vi "Data entry form multi-module.vi"(8 "error in (no error)":errorcluster, 9 "Assembly Type":string, 10 "Is Module?":bool, 11 "Database Entry in":refnum<class "Database Entry.lvclass">) -> (0 "error out":errorcluster, 1 "Is Dummy run?":bool, 2 "Aborted":bool, 3 "Database Entry out":refnum<class "Database Entry.lvclass">)   [LabVIEW 2021, in "Database Entry.lvclass"]
uses:
  Database Entry.lvclass
  Database Entry.lvclass/Database Entry.ctl
  Components/Stack/Stack.lvclass
panel:
  out "RingText.Text":string
  out "Now assembling...":string
  in  "Protomodule Steps":T1(ring)
  in  "Module Steps":T2(ring)
  in  "Dummy run submit":bool
  out "Use same values for both":bool
  in  "Use same values for all":bool
  out "Instructions":string
  in  "Module Instuctions":T3(ring)
  in  "Protomodule Instructions":T4(ring)
  in  "Submit":bool
  in  "Gantry":T5
  out "Stage":string
  in  "Steps":T6(ring)
  in  "Abort":bool
  in  "Next":bool
  in  "Previous":bool
  # "Col 1"
  # "Col 2"
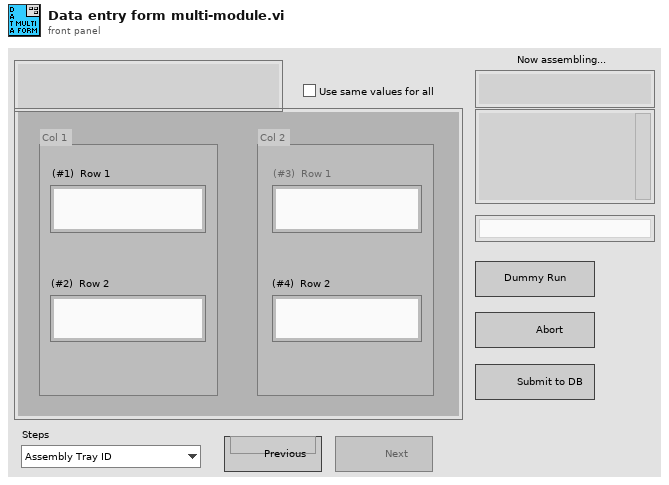
[diagram p1: front panel]
types:
  T1 = enum16{"Assembly Tray ID", "Module Stack ID", "Baseplate ID", "Sensor PUT ID", "Sensor Tray ID", "Sensor ID", "Sensor grade", "Comments", "Glue batch number", "Tape batch number"}
  T2 = enum16{"Assembly Tray ID", "Module Stack ID", "Protomodule ID", "Hexaboard PUT ID", "Hexaboard Tray ID", "Hexaboard ID", "Sensor grade", "Comments", "Glue batch number", "Tape batch number"}
  T3 = enum16{"Assembly Tray ID is always required.                For dummy runs, skip entry of other data.", "Scan the MODULE QR code (320M).                 **Leave blank for dummy runs**", "Verify the protomodule ID (320P) or scan the module QR code.                 **Leave blank for dummy runs**", "Hexaboard pick-up-tool ID", "Hexaboard Tray ID", "Scan the hexaboard QR code (320XL).                 **Leave blank for dummy runs**", "(Optional) Leave blank if no updated grade for the sensor", "Comments, if any.", "Glue batch number", "Tape batch number"}
  T4 = enum16{"Assembly Tray ID is always required.                For dummy runs, skip entry of other data.", "Scan the MODULE QR code (320M) for this protomodule.                 **Leave blank for dummy runs**", "Scan the baseplate QR code (320BA).                 **Leave blank for dummy runs**", "Sensor pick-up-tool ID", "Sensor Tray ID", "Scan the sensor barcode.                 **Leave blank for dummy runs**", "Sensor grade (default A)", "Include sensor visual inspection comments here.", "Glue batch number", "(Optional) Tape batch number"}
  T5 = cluster{"(#1)  Row 1":string, "(#2)  Row 2":string, "(#3)  Row 1":string, "(#4)  Row 2":string}
  T6 = enum16{"Assembly Tray ID", "Module Stack ID", "Base-layer (BP/PL) ID", "Pick-up-tool ID", "Component Tray ID", "Top-layer (Sen/Hxb) ID", "Sensor grade", "Comments", "Glue batch number"}
  T7 = enum8{"Enabled", "Disabled", "Disabled and Grayed Out"}
  T8 = enum16{"Assembly Tray ID", "Module Stack ID", "Base-layer (BP/PL) ID", "Pick-up-tool ID", "Component Tray ID", "Top-layer (Sen/Hxb) ID", "Sensor grade", "Comments", "Glue batch number", "Tape batch number"}
  T9 = cluster{"(#1)  Pos 1":string, "(#2)  Pos 2":string, "(#3)  Pos 1":string, "(#4)  Pos 2":string}
  T10 = cluster{"Value[0]":string, "Value[1]":string, "Value[2]":string, "Value[3]":string}
  T11 = cluster{"[0]":string, "[1]":string, "[2]":string, "[3]":string}
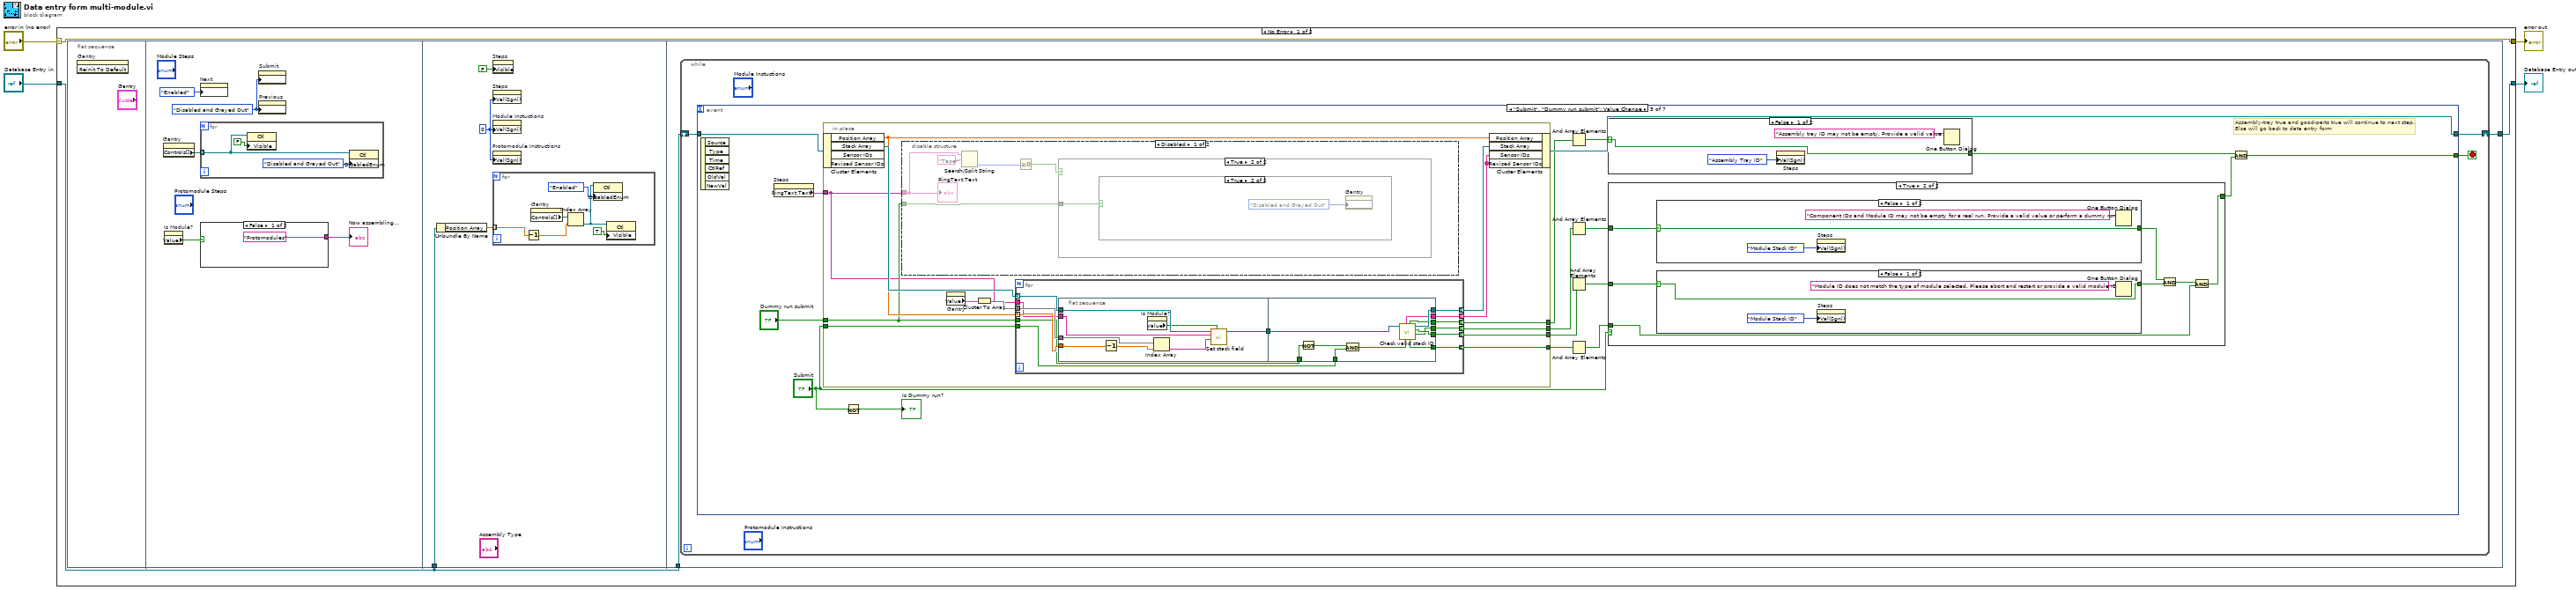
[diagram p0: block diagram]
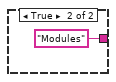
[diagram p2: hidden frame]
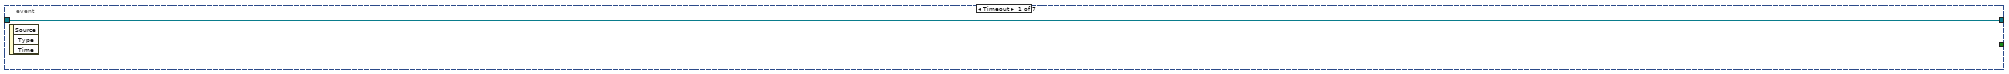
[diagram p3: hidden frame]
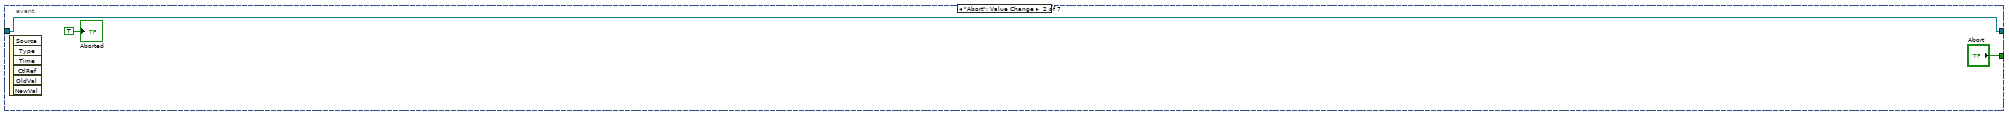
[diagram p4: hidden frame]
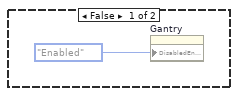
[diagram p5: hidden frame]
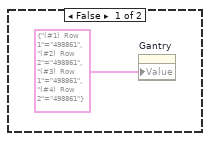
[diagram p6: hidden frame]
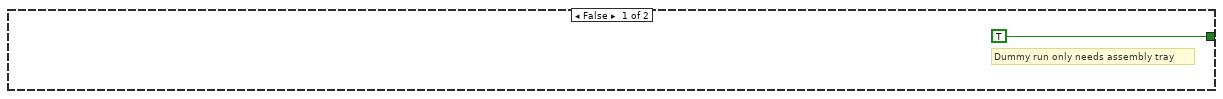
[diagram p8: hidden frame]
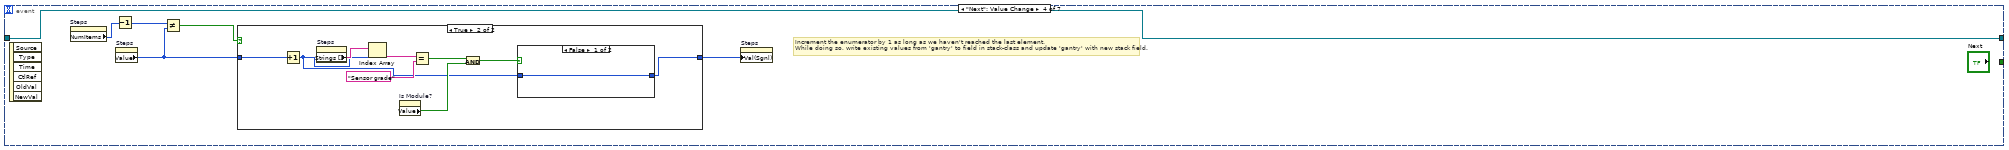
[diagram p12: hidden frame]
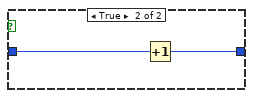
[diagram p14: hidden frame]
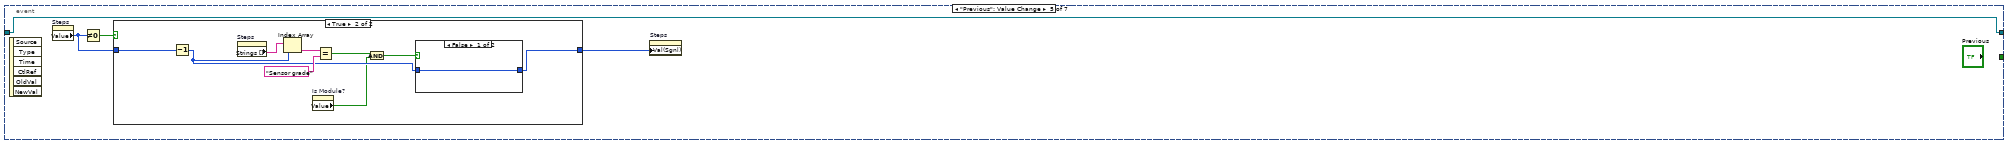
[diagram p15: hidden frame]
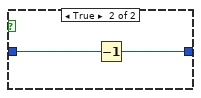
[diagram p17: hidden frame]
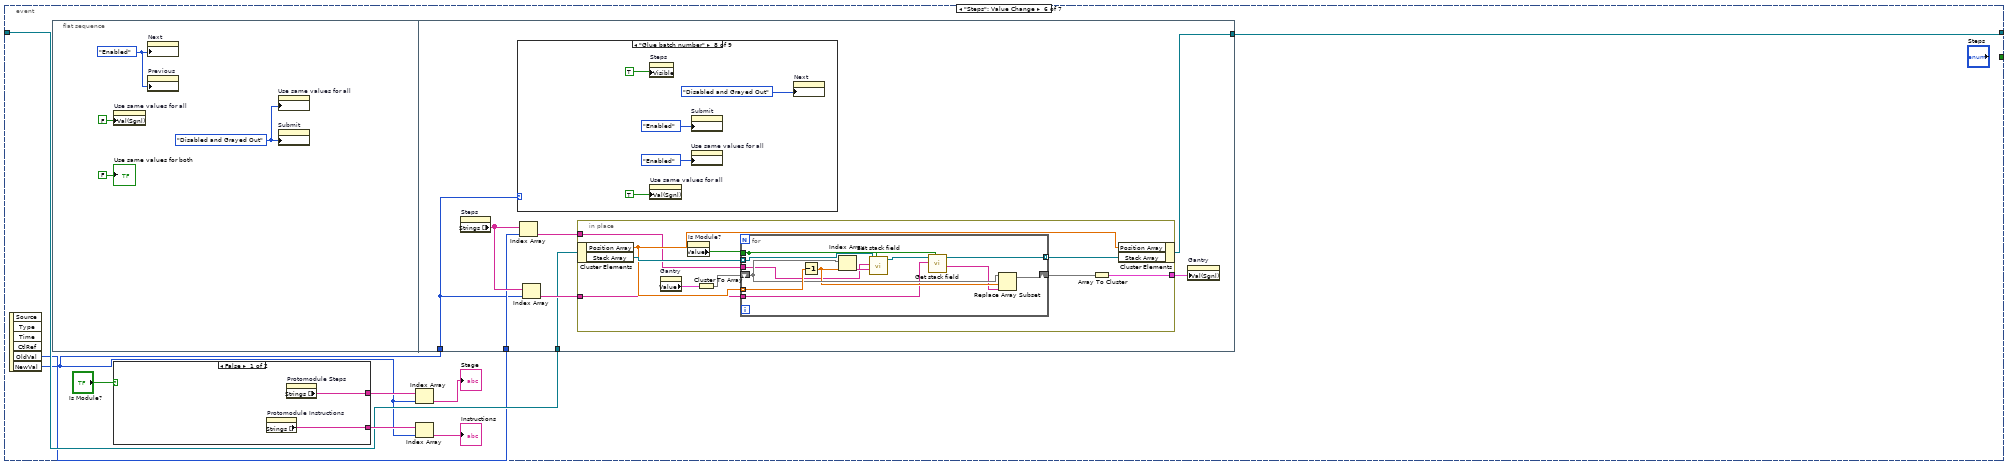
[diagram p18: hidden frame]
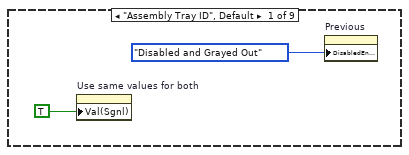
[diagram p19: hidden frame]
diagram:
  n1 = case shown="No Error" "error in (no error)" {
    selector: "error in (no error)" -> [w7 w301]
    tunnel: [w7 w301] -> w3
    tunnel: "Database Entry in" -> [w5 w300]
    tunnel: [w6 w300] -> w1
    frame No Error {
      n2 = flat-sequence {
        tunnel: w5 -> [w19]
        tunnel: w5 -> [w28]
        tunnel: [w29] -> w6
        frame #0 {
          n3 = invoke on="Gantry" class="Clust (strict)" method="Reinit To Default"() -> ()  [unwired: 3 in, 3 out]
        }
        frame #1 {
          w11 = T7."Disabled and Grayed Out" ("Disabled")
          n4 = property on="Gantry" class="Clust (strict)"() -> ("Controls[]"=w12:refnum<vi>[])  [unwired: 2 in, 2 out]
          n5 = property on="Is Module?" class="Bool (strict)"() -> ("Value"=w8:bool)  [unwired: 2 in, 2 out]
          n6 = property on="Next" class="Bool"("DisabledEnum"=T7."Enabled" ("Disabled")) -> ()  [unwired: 2 in, 2 out]
          n7 = for {
            tunnel: w12 -> [w15] mode=indexing
            n8 = property class="Ctl"(reference=w15, "Visible"=FALSE) -> ()  [unwired: 1 in, 2 out]
            n9 = property class="Ctl"(reference=w15, "DisabledEnum"=T7."Disabled and Grayed Out" ("Disabled")) -> ()  [unwired: 1 in, 2 out]
          }
          n10 = case shown="False" w8 {
            tunnel: ["Protomodules" ("Now assembling...") "Modules" ("Now assembling...")] -> w9
            frame False {
            }
            frame True {
            }
          }
          "Now assembling..." <- w9
          n11 = property on="Submit" class="Bool"("DisabledEnum"=w11) -> ()  [unwired: 2 in, 2 out]
          n12 = property on="Previous" class="Bool"("DisabledEnum"=w11) -> ()  [unwired: 2 in, 2 out]
        }
        frame #2 {
          w20 = u16 0 ("Value (Signaling)")
          n13 = Unbundle By Name(w19) -> ("Position Array"=w18:dbl[])
          n14 = property on="Steps" class="Enum (strict)"("Visible"=FALSE) -> ()  [unwired: 2 in, 2 out]
          n15 = property on="Steps" class="Enum (strict)"("Val(Sgnl)"=w20) -> ()  [unwired: 2 in, 2 out]
          n16 = property on="Module Instuctions" class="Enum (strict)"("Val(Sgnl)"=w20) -> ()  [unwired: 2 in, 2 out]
          n17 = property on="Protomodule Instructions" class="Enum (strict)"("Val(Sgnl)"=w20) -> ()  [unwired: 2 in, 2 out]
          n18 = for {
            tunnel: w18 -> [w23] mode=indexing
            n19 = Decrement(x=w23) -> (x-1=w22:dbl)
            n20 = property on="Gantry" class="Clust (strict)"() -> ("Controls[]"=w27:refnum<vi>[])  [unwired: 2 in, 2 out]
            n21 = Index Array(array=w27, index=w22) -> (element=w25:refnum<vi>)
            n22 = property class="Ctl"(reference=w25, "DisabledEnum"=T7."Enabled" ("Disabled")) -> ()  [unwired: 1 in, 2 out]
            n23 = property class="Ctl"(reference=w25, "Visible"=TRUE) -> ()  [unwired: 1 in, 2 out]
          }
        }
        frame #3 {
          n24 = while {
            shift-right: [w31] -> w29
            shift-left: w28 -> [w30]
            stop <- w32 stop-if-true
            # "While loop"
            n25 = event shown="[2] \"Submit\", \"Dummy run submit\": Value Change" {
              selector: _ -> [_ _ _ _ _ _ _]
              dyn-events: _ -> [_ _ _ _ _ _ _]
              timeout: _ -> [_ _ _ _ _ _ _]
              tunnel: [_ "Abort" w42 _ _ _ _] -> w32
              tunnel: w30 -> [w33 w35 w53 w128 w147 w167 w219]
              tunnel: [w33 w35 w52 w128 w147 w166 w219] -> w31
              event Timeout {
                n26 = event-data() -> ()  [unwired: 1 in, 3 out]
              }
              event "Abort": Value Change {
                n27 = event-data() -> ()  [unwired: 1 in, 6 out]
                "Aborted" <- TRUE ("Aborted")
              }
              event "Submit", "Dummy run submit": Value Change {
                # "Assembly-tray true and good-parts true will continue to next step. \nElse will go back to data entry form"
                n28 = event-data() -> ()  [unwired: 1 in, 6 out]
                n29 = property on="Steps" class="Enum (strict)"() -> ("RingText.Text"=w48:string)  [unwired: 2 in, 2 out]
                n30 = in-place {
                  in-place-border: w48 -> [w55]
                  in-place-border: [w61] -> w51
                  in-place-border: [w60] -> w50
                  in-place-border: [w59] -> w49
                  in-place-border: "Dummy run submit" -> [w58]
                  in-place-border: "Submit" -> [w57]
                  in-place-border: [w56] -> w38
                  n31 = in-place-cluster #1(w53) -> ("Position Array"=w65:dbl[], "Stack Array"=w66:refnum<class "Stack.lvclass">[])  [unwired: 2 out]
                  n32 = disable-structure shown="Disabled" {
                    disable-tunnel: w58 -> [w71 _]
                    disable-tunnel: w55 -> [w70 _]
                    frame Disabled {
                      n33 = Search/Split String(string=w70, search string/char (-)="Tape") -> (offset of match=w68:i32)  [unwired: 1 in, 2 out]
                      n34 = Greater Or Equal To 0?(x=w68) -> (x >= 0?=w67:bool)
                      n35 = case shown="True" w67 {
                        tunnel: w71 -> [_ w73]
                        frame False {
                          n36 = property on="Gantry" class="Clust (strict)"("DisabledEnum"=T7."Enabled" ("Disabled")) -> ()  [unwired: 2 in, 2 out]
                        }
                        frame True {
                          n37 = case shown="True" w73 {
                            frame False {
                              n38 = property on="Gantry" class="Clust (strict)"("Value"=T5 {"(#1)  Row 1"="498861", "(#2)  Row 2"="498861", "(#3)  Row 1"="498861", "(#4)  Row 2"="498861"} ("Gantry")) -> ()  [unwired: 2 in, 2 out]
                            }
                            frame True {
                              n39 = property on="Gantry" class="Clust (strict)"("DisabledEnum"=T7."Disabled and Grayed Out" ("Disabled")) -> ()  [unwired: 2 in, 2 out]
                            }
                          }
                        }
                      }
                      "RingText.Text" <- w70
                    }
                    frame Enabled {
                    }
                  }
                  n40 = property on="Gantry" class="Clust (strict)"() -> ("Value"=w63:T9)  [unwired: 2 in, 2 out]
                  n41 = Cluster To Array(cluster=w63) -> (array=w64:string[])
                  n42 = for {
                    tunnel: w66 -> [w88] mode=indexing
                    tunnel: w65 -> [w87] mode=indexing
                    tunnel: [w85] -> w62 mode=indexing
                    tunnel: w55 -> [w78]
                    tunnel: w64 -> [w86]
                    tunnel: w57 -> [w83]
                    tunnel: w58 -> [w77]
                    tunnel: [w82] -> w61 mode=indexing
                    tunnel: [w81] -> w60 mode=indexing
                    tunnel: [w80] -> w59 mode=indexing
                    tunnel: [w79] -> w56 mode=indexing
                    tunnel: [w76] -> w54 mode=indexing
                    n43 = flat-sequence {
                      tunnel: w88 -> [w96]
                      tunnel: w87 -> [w95]
                      tunnel: w86 -> [w93]
                      tunnel: w78 -> [w91]
                      tunnel: [w90] -> w84
                      tunnel: [w106] -> w85
                      tunnel: w84 -> [w107]
                      tunnel: w83 -> [w104]
                      tunnel: w77 -> [w103]
                      tunnel: [w101] -> w82
                      tunnel: [w100] -> w81
                      tunnel: [w99] -> w80
                      tunnel: [w98] -> w79
                      tunnel: [w97] -> w76
                      frame #0 {
                        n44 = Decrement(x=w95) -> (x-1=w92:dbl)
                        n45 = property on="Is Module?" class="Bool (strict)"() -> ("Value"=w89:bool)  [unwired: 2 in, 2 out]
                        n46 = Index Array(array=w93, index=w92) -> (element=w94:string)
                        n47 = call "Set stack field.vi"("Is Module?"=w89, "Value in"=w94, "Field"=w91, "Stack in"=w96) -> ("Stack out"=w90:refnum<class "Stack.lvclass">)  [unwired: 6 in, 1 out]
                      }
                      frame #1 {
                        n48 = Not(x=w103) -> (.not. x?=w102:bool)
                        n49 = And(x=w102, y=w104) -> (x .and. y?=w105:bool)
                        n50 = call "Check valid stack ID.vi"("Is real run?"=w105, "Stack in"=w107) -> ("Non-empty part IDs?"=w100:bool, "Valid module ID?"=w101:bool, "Stack out"=w106:refnum<class "Stack.lvclass">, "Continue with current parts"=w98:bool, "Non-empty assembly tray ID?"=w99:bool, "Sensor ID out"=w97:string)  [unwired: 3 in, 1 out]
                      }
                    }
                  }
                  n51 = in-place-cluster #1("Position Array"=w65, "Stack Array"=w62, "Sensor IDs"=w54, "Revised Sensor IDs"=w54) -> (w52:refnum<class "Database Entry.lvclass">)
                }
                n52 = Not(x="Submit") -> (.not. x?=→"Is Dummy run?":bool)
                n53 = And Array Elements(Boolean array=w49) -> (logical AND=w47:bool)
                n54 = And Array Elements(Boolean array=w50) -> (logical AND=w46:bool)
                n55 = And Array Elements(Boolean array=w51) -> (logical AND=w44:bool)
                n56 = And Array Elements(Boolean array=w38) -> (logical AND=w37:bool)
                n57 = case shown="False" w47 {
                  selector: w47 -> [w125 w127]
                  tunnel: [w125 w127] -> w43
                  frame False {
                    n58 = property on="Steps" class="Enum (strict)"("Val(Sgnl)"=T8."Assembly Tray ID" ("Value (Signaling)")) -> ()  [unwired: 2 in, 2 out]
                    n59 = One Button Dialog(message="Assembly tray ID may not be empty. Provide a valid value.") -> ()  [unwired: 1 in, 1 out]
                  }
                  frame True {
                  }
                }
                n60 = case shown="True" "Submit" {
                  tunnel: w46 -> [_ w115]
                  tunnel: w44 -> [_ w114]
                  tunnel: [TRUE w109] -> w41
                  tunnel: w37 -> [_ w111]
                  frame False {
                    # "Dummy run only needs assembly tray"
                  }
                  frame True {
                    n61 = case shown="False" w115 {
                      selector: w115 -> [w121 w123]
                      tunnel: [w121 w123] -> w113
                      frame False {
                        n62 = property on="Steps" class="Enum (strict)"("Val(Sgnl)"=T8."Module Stack ID" ("Value (Signaling)")) -> ()  [unwired: 2 in, 2 out]
                        n63 = One Button Dialog(message="Component IDs and Module ID may not be empty for a real run. Provide a valid value or perform a dummy run.") -> ()  [unwired: 1 in, 1 out]
                      }
                      frame True {
                      }
                    }
                    n64 = case shown="False" w114 {
                      selector: w114 -> [w117 w119]
                      tunnel: [w117 w119] -> w112
                      frame False {
                        n65 = property on="Steps" class="Enum (strict)"("Val(Sgnl)"=T8."Module Stack ID" ("Value (Signaling)")) -> ()  [unwired: 2 in, 2 out]
                        n66 = One Button Dialog(message="Module ID does not match the type of module selected. Please abort and restart or provide a valid module ID.") -> ()  [unwired: 1 in, 1 out]
                      }
                      frame True {
                      }
                    }
                    n67 = And(x=w113, y=w112) -> (x .and. y?=w110:bool)
                    n68 = And(x=w110, y=w111) -> (x .and. y?=w109:bool)
                  }
                }
                n69 = And(x=w43, y=w41) -> (x .and. y?=w42:bool)
              }
              event "Next": Value Change {
                # "Increment the enumerator by 1 as long as we haven't reached the last element.\nWhile doing so, write existing values from 'gantry' to field in stack-class and update 'gantry' with new stack field."
                n70 = event-data() -> ()  [unwired: 1 in, 6 out]
                n71 = property on="Steps" class="Enum (strict)"() -> ("NumItems"=w133:u32)  [unwired: 2 in, 2 out]
                n72 = Decrement(x=w133) -> (x-1=w132:u32)
                n73 = property on="Steps" class="Enum (strict)"() -> ("Value"=w130:T6)  [unwired: 2 in, 2 out]
                n74 = Not Equal?(x=w132, y=w130) -> (x != y?=w131:bool)
                n75 = case shown="True" w131 {
                  tunnel: w130 -> [w134 w143]
                  tunnel: [w134 w135] -> w129
                  frame False {
                  }
                  frame True {
                    n76 = Increment(x=w143) -> (x+1=w136:T6)
                    n77 = property on="Steps" class="Enum (strict)"() -> ("Strings []"=w142:string[])  [unwired: 2 in, 2 out]
                    n78 = Index Array(array=w142, index=w136) -> (element=w141:string)
                    n79 = property on="Is Module?" class="Bool (strict)"() -> ("Value"=w138:bool)  [unwired: 2 in, 2 out]
                    n80 = Equal?(x=w141, y="Sensor grade") -> (x = y?=w139:bool)
                    n81 = And(x=w139, y=w138) -> (x .and. y?=w137:bool)
                    n82 = case shown="False" w137 {
                      tunnel: w136 -> [w144 w146]
                      tunnel: [w144 w145] -> w135
                      frame False {
                      }
                      frame True {
                        n83 = Increment(x=w146) -> (x+1=w145:T6)
                      }
                    }
                  }
                }
                n84 = property on="Steps" class="Enum (strict)"("Val(Sgnl)"=w129) -> ()  [unwired: 2 in, 2 out]
              }
              event "Previous": Value Change {
                n85 = event-data() -> ()  [unwired: 1 in, 6 out]
                n86 = property on="Steps" class="Enum (strict)"() -> ("Value"=w149:T6)  [unwired: 2 in, 2 out]
                n87 = Not Equal To 0?(x=w149) -> (x != 0?=w150:bool)
                n88 = case shown="True" w150 {
                  tunnel: w149 -> [w151 w160]
                  tunnel: [w151 w152] -> w148
                  frame False {
                  }
                  frame True {
                    n89 = Decrement(x=w160) -> (x-1=w155:T6)
                    n90 = property on="Steps" class="Enum (strict)"() -> ("Strings []"=w154:string[])  [unwired: 2 in, 2 out]
                    n91 = Index Array(array=w154, index=w155) -> (element=w159:string)
                    n92 = property on="Is Module?" class="Bool (strict)"() -> ("Value"=w153:bool)  [unwired: 2 in, 2 out]
                    n93 = Equal?(x=w159, y="Sensor grade") -> (x = y?=w157:bool)
                    n94 = And(x=w157, y=w153) -> (x .and. y?=w156:bool)
                    n95 = case shown="False" w156 {
                      tunnel: w155 -> [w161 w163]
                      tunnel: [w161 w162] -> w152
                      frame False {
                      }
                      frame True {
                        n96 = Decrement(x=w163) -> (x-1=w162:T6)
                      }
                    }
                  }
                }
                n97 = property on="Steps" class="Enum (strict)"("Val(Sgnl)"=w148) -> ()  [unwired: 2 in, 2 out]
              }
              event "Steps": Value Change {
                n98 = event-data() -> ("OldVal"=w165:T6, "NewVal"=w164:T6)  [unwired: 1 in, 4 out]
                n99 = flat-sequence {
                  tunnel: [w179] -> w166
                  tunnel: w167 -> [w180]
                  tunnel: w165 -> [w178]
                  tunnel: w164 -> [w177]
                  frame #0 {
                    w176 = T7."Disabled and Grayed Out" ("Disabled")
                    w175 = T7."Enabled" ("Disabled")
                    n100 = property on="Use same values for all" class="Bool (strict)"("Val(Sgnl)"=FALSE ("Value (Signaling)")) -> ()  [unwired: 2 in, 2 out]
                    n101 = property on="Next" class="Bool"("DisabledEnum"=w175) -> ()  [unwired: 2 in, 2 out]
                    n102 = property on="Previous" class="Bool"("DisabledEnum"=w175) -> ()  [unwired: 2 in, 2 out]
                    n103 = property on="Use same values for all" class="Bool (strict)"("DisabledEnum"=w176) -> ()  [unwired: 2 in, 2 out]
                    n104 = property on="Submit" class="Bool"("DisabledEnum"=w176) -> ()  [unwired: 2 in, 2 out]
                    "Use same values for both" <- FALSE ("Use same values for both")
                  }
                  frame #1 {
                    n105 = property on="Steps" class="Enum (strict)"() -> ("Strings []"=w181:string[])  [unwired: 2 in, 2 out]
                    n106 = case shown="\"Glue batch number\"" w177 {
                      frame "Assembly Tray ID", Default {
                        n107 = property on="Use same values for both" class="Bool (strict)"("Val(Sgnl)"=TRUE ("Value (Signaling)")) -> ()  [unwired: 2 in, 2 out]
                        n108 = property on="Previous" class="Bool"("DisabledEnum"=T7."Disabled and Grayed Out" ("Disabled")) -> ()  [unwired: 2 in, 2 out]
                      }
                      frame "Module Stack ID" {
                      }
                      frame "Base-layer (BP/PL) ID" {
                      }
                      frame "Pick-up-tool ID" {
                      }
                      frame "Component Tray ID" {
                        n109 = property on="Use same values for both" class="Bool (strict)"("Val(Sgnl)"=TRUE ("Value (Signaling)")) -> ()  [unwired: 2 in, 2 out]
                      }
                      frame "Top-layer (Sen/Hxb) ID" {
                      }
                      frame "Comments" {
                      }
                      frame "Glue batch number" {
                        n110 = property on="Steps" class="Enum (strict)"("Visible"=TRUE) -> ()  [unwired: 2 in, 2 out]
                        n111 = property on="Use same values for all" class="Bool (strict)"("Val(Sgnl)"=TRUE ("Value (Signaling)")) -> ()  [unwired: 2 in, 2 out]
                        n112 = property on="Submit" class="Bool"("DisabledEnum"=T7."Enabled" ("Disabled")) -> ()  [unwired: 2 in, 2 out]
                        n113 = property on="Use same values for all" class="Bool (strict)"("DisabledEnum"=T7."Enabled" ("Disabled")) -> ()  [unwired: 2 in, 2 out]
                        n114 = property on="Next" class="Bool"("DisabledEnum"=T7."Disabled and Grayed Out" ("Disabled")) -> ()  [unwired: 2 in, 2 out]
                      }
                      frame "Sensor grade" {
                      }
                    }
                    n115 = Index Array(array=w181, index=w178) -> (element=w182:string)
                    n116 = Index Array(array=w181, index=w177) -> (element=w183:string)
                    n117 = in-place {
                      in-place-border: w182 -> [w198]
                      in-place-border: w183 -> [w197]
                      in-place-border: [w193] -> w184
                      n118 = in-place-cluster #2(w180) -> ("Position Array"=w201:dbl[], "Stack Array"=w202:refnum<class "Stack.lvclass">[])
                      n119 = property on="Gantry" class="Clust (strict)"() -> ("Value"=w196:T9)  [unwired: 2 in, 2 out]
                      n120 = property on="Is Module?" class="Bool (strict)"() -> ("Value"=w195:bool)  [unwired: 2 in, 2 out]
                      n121 = Cluster To Array(cluster=w196) -> (array=w199:string[])
                      n122 = for {
                        tunnel: w202 -> [w214] mode=indexing
                        tunnel: w201 -> [w213] mode=indexing
                        tunnel: [w212] -> w200 mode=indexing
                        tunnel: w198 -> [w205]
                        tunnel: w197 -> [w204]
                        tunnel: w195 -> [w203]
                        shift-right: [w206] -> w194
                        shift-left: w199 -> [w209]
                        n123 = Decrement(x=w213) -> (x-1=w208:dbl)
                        n124 = Index Array(array=w209, index=w208) -> (element=w210:string)
                        n125 = call "Set stack field.vi"("Is Module?"=w203, "Value in"=w210, "Field"=w205, "Stack in"=w214) -> ("Stack out"=w211:refnum<class "Stack.lvclass">)  [unwired: 6 in, 1 out]
                        n126 = call "Get stack field.vi"("Is Module?"=w203, "Field"=w204, "Stack in"=w211) -> ("Value out"=w207:string, "Stack out"=w212:refnum<class "Stack.lvclass">)  [unwired: 6 in, 1 out]
                        n127 = Replace Array Subset(array=w209, new element=w207, index=w208) -> (w206:string[])
                      }
                      n128 = Array To Cluster(array=w194) -> (cluster=w193:T10)
                      n129 = in-place-cluster #2("Position Array"=w201, "Stack Array"=w200) -> (w179:refnum<class "Database Entry.lvclass">)
                    }
                    n130 = property on="Gantry" class="Clust (strict)"("Val(Sgnl)"=w184) -> ()  [unwired: 2 in, 2 out]
                  }
                }
                n131 = case shown="False" "Is Module?" {
                  tunnel: [w216 w218] -> w172
                  tunnel: [w215 w217] -> w168
                  frame False {
                    n132 = property on="Protomodule Instructions" class="Enum (strict)"() -> ("Strings []"=w216:string[])  [unwired: 2 in, 2 out]
                    n133 = property on="Protomodule Steps" class="Enum (strict)"() -> ("Strings []"=w215:string[])  [unwired: 2 in, 2 out]
                  }
                  frame True {
                    n134 = property on="Module Instuctions" class="Enum (strict)"() -> ("Strings []"=w218:string[])  [unwired: 2 in, 2 out]
                    n135 = property on="Module Steps" class="Enum (strict)"() -> ("Strings []"=w217:string[])  [unwired: 2 in, 2 out]
                  }
                }
                n136 = Index Array(array=w168, index=w164) -> (element=→"Stage":string)
                n137 = Index Array(array=w172, index=w164) -> (element=→"Instructions":string)
              }
              event "Gantry": Value Change {
                n138 = event-data() -> ("OldVal"=w222:T5, "NewVal"=w221:T5)  [unwired: 1 in, 4 out]
                n139 = property on="Use same values for both" class="Bool (strict)"() -> ("Value"=w220:bool)  [unwired: 2 in, 2 out]
                n140 = case shown="False" "Use same values for all" {
                  tunnel: w221 -> [_ w284]
                  tunnel: w222 -> [_ w282]
                  frame False {
                  }
                  frame True {
                    # "If all strings have same value, do nothing. If false, make them same."
                    n141 = Cluster To Array(cluster=w282) -> (array=w283:string[])
                    n142 = Cluster To Array(cluster=w284) -> (array=w281:string[])
                    n143 = Index Array(array=w281) -> (element=w280:string)  [unwired: 1 in]
                    n144 = Equal?(x=w281, y=w280) -> (x = y?=w279:bool[])
                    n145 = And Array Elements(Boolean array=w279) -> (logical AND=w278:bool)
                    n146 = case shown="False" w278 {
                      tunnel: w283 -> [w291 _]
                      tunnel: w281 -> [w288 _]
                      frame False {
                        n147 = Not Equal?(x=w291, y=w288) -> (x != y?=w294:bool[])
                        n148 = Array Size(array=w288) -> (size(s)=w290:i32)
                        n149 = Search 1D Array(1D array=w294, element=TRUE) -> (index of element=w293:i32)  [unwired: 1 in]
                        n150 = Index Array(array=w288, index=w293) -> (element=w292:string)
                        n151 = for {
                          N: w290 -> [_]
                          tunnel: w292 -> [w297]
                          shift-right: [w298] -> w287
                          shift-left: string[] [] -> [w296]
                          i -> [w299]
                          n152 = Insert Into Array(array=w296, index=w299, new element=w297) -> (w298:string[])
                        }
                        n153 = Array Subset(array=w287, length=w290) -> (w286:string[])  [unwired: 1 in]
                        n154 = Array To Cluster(array=w286) -> (cluster=w289:T11)
                        n155 = property on="Gantry" class="Clust (strict)"("Val(Sgnl)"=w289) -> ()  [unwired: 2 in, 2 out]
                      }
                      frame True {
                      }
                    }
                  }
                }
                n156 = case shown="True" w220 {
                  tunnel: w221 -> [_ w232]
                  tunnel: w222 -> [_ w231]
                  frame False {
                  }
                  frame True {
                    # "no of trays"
                    n157 = Cluster To Array(cluster=w231) -> (array=w226:string[])
                    n158 = Cluster To Array(cluster=w232) -> (array=w225:string[])
                    n159 = Array Size(array=w225) -> (size(s)=w230:i32)
                    n160 = Divide(x=w230, y=2) -> (x/y=w228:dbl)
                    n161 = for {
                      N: w228 -> [_]
                      tunnel: w225 -> [w237]
                      tunnel: [w236] -> w224 mode=indexing
                      i -> [w235]
                      # "The two positions in a given tray have same tray id value. If false, set them to have same value"
                      n162 = Multiply(x=2 ("y"), y=w235) -> (x*y=w233:i32)
                      n163 = Increment(x=w233) -> (x+1=w240:i32)
                      n164 = Index Array(array=w237, index #1=w233, index #2=w240) -> (element #1=w238:string, element #2=w239:string)
                      n165 = Equal?(x=w238, y=w239) -> (x = y?=w236:bool)
                    }
                    n166 = And Array Elements(Boolean array=w224) -> (logical AND=w227:bool)
                    n167 = case shown="True" w227 {
                      tunnel: w226 -> [w244 _]
                      tunnel: w225 -> [w248 _]
                      tunnel: w228 -> [w249 _]
                      tunnel: w224 -> [w241 _]
                      frame False {
                        n168 = Array Size(array=w244) -> (size(s)=w245:i32)
                        n169 = for {
                          N: w249 -> [_]
                          tunnel: w244 -> [w255]
                          tunnel: w248 -> [w253]
                          shift-right: [w251] -> w246
                          shift-left: string[] [] -> [w252]
                          tunnel: w241 -> [w250] mode=indexing
                          i -> [w254]
                          # "If the two positions in a tray have diff values, make them same. Else retain original values"
                          n170 = case shown="True" w250 {
                            tunnel: w255 -> [w268 _]
                            tunnel: w254 -> [w267 w274]
                            tunnel: w253 -> [w266 w275]
                            tunnel: w252 -> [w259 w273]
                            tunnel: [w258 w270] -> w251
                            frame False {
                              w265 = 2 ("length")
                              n171 = Multiply(x=2 ("y"), y=w267) -> (x*y=w257:i32)
                              n172 = Array Subset(array=w268, index=w257, length=w265) -> (w264:string[])
                              n173 = Array Subset(array=w266, index=w257, length=w265) -> (w261:string[])
                              n174 = Not Equal?(x=w264, y=w261) -> (x != y?=w263:bool[])
                              n175 = Search 1D Array(1D array=w263, element=TRUE) -> (index of element=w260:i32)  [unwired: 1 in]
                              n176 = Index Array(array=w261, index=w260) -> (element=w256:string)
                              n177 = Insert Into Array(array=w259, index=w257, new element #1=w256, new element #2=w256) -> (w258:string[])
                            }
                            frame True {
                              n178 = Multiply(x=2 ("y"), y=w274) -> (x*y=w272:i32)
                              n179 = Array Subset(array=w275, index=w272, length=2) -> (w271:string[])
                              n180 = Insert Into Array(array=w273, index=w272, new element=w271) -> (w270:string[])
                            }
                          }
                        }
                        n181 = Array Subset(array=w246, length=w245) -> (w243:string[])  [unwired: 1 in]
                        n182 = Array To Cluster(array=w243) -> (cluster=w242:T11)
                        n183 = property on="Gantry" class="Clust (strict)"("Val(Sgnl)"=w242) -> ()  [unwired: 2 in, 2 out]
                      }
                      frame True {
                      }
                    }
                  }
                }
              }
            }
          }
        }
      }
    }
    frame Error {
    }
  }
  "error out" <- w3
  "Database Entry out" <- w1
